vi "导轨命令.vi"(8 "error in":errorcluster, 9 "执行程序零":bool, 10 "绝对位置":i32, 11 "速度":i32) -> (0 "error out":errorcluster, 3 "输出字符串":string)   [LabVIEW 2016]
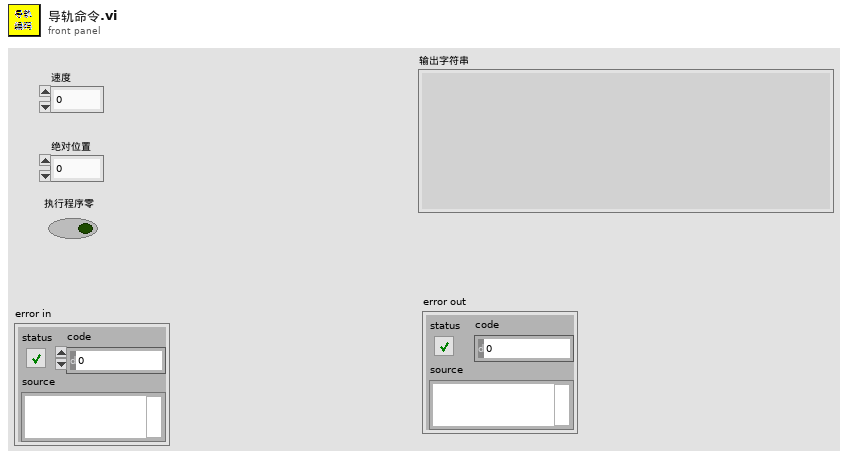
[diagram p1: front panel]
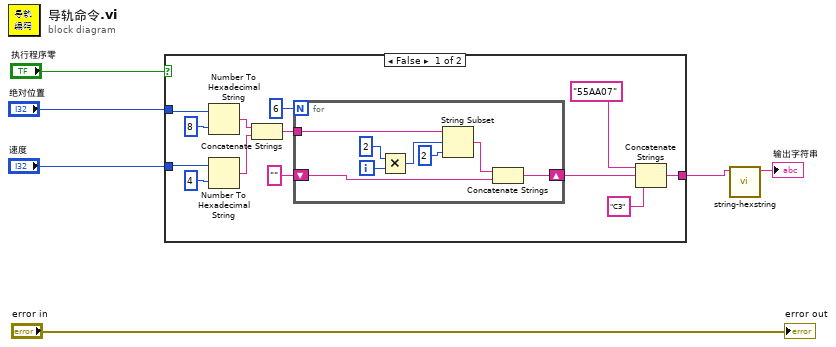
[diagram p0: block diagram]
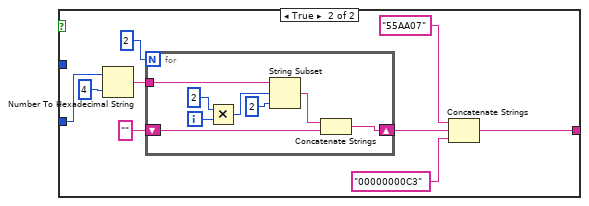
[diagram p2: hidden frame]
diagram:
  n1 = case shown="False" "执行程序零" {
    tunnel: "绝对位置" -> [w9 _]
    tunnel: "速度" -> [w8 w29]
    tunnel: [w7 w28] -> w3
    frame False {
      n2 = Number To Hexadecimal String(1:i16 8 ("width (-)"), 2:w9) -> (0:w19:string)
      n3 = Number To Hexadecimal String(1:i16 4 ("width (-)"), 2:w8) -> (0:w18:string)
      n4 = Concatenate Strings(w19, w18) -> (w17:string)
      n5 = for {
        N: 6 -> [_]
        shift-right: [w23] -> w13
        shift-left: "" -> [w21]
        tunnel: w17 -> [w22]
        i -> [w27]
        n6 = Multiply(x=2, y=w27) -> (x*y=w24:i32)
        n7 = String Subset(string=w22, offset (0)=w24, length (rest)=2 ("length (rest)")) -> (substring=w20:string)
        n8 = Concatenate Strings(w20, w21) -> (w23:string)
      }
      n9 = Concatenate Strings("55AA07" ("string"), w13, "C3" ("string")) -> (w7:string)
    }
    frame True {
      n10 = Number To Hexadecimal String(1:i16 4 ("width (-)"), 2:w29) -> (0:w33:string)
      n11 = for {
        N: 2 -> [_]
        shift-right: [w40] -> w36
        shift-left: "" -> [w38]
        tunnel: w33 -> [w39]
        i -> [w44]
        n12 = Multiply(x=2, y=w44) -> (x*y=w41:i32)
        n13 = String Subset(string=w39, offset (0)=w41, length (rest)=2 ("length (rest)")) -> (substring=w37:string)
        n14 = Concatenate Strings(w37, w38) -> (w40:string)
      }
      n15 = Concatenate Strings("55AA07" ("string"), w36, "00000000C3" ("string")) -> (w28:string)
    }
  }
  n16 = call "string-hexstring.vi"("字符串"=w3) -> ("十六进制整型字符串"=→"输出字符串":string)  [unwired: 10 in]
  "error out" <- "error in"
